vi "Delacor_lib_QMH_Error Handler - Message Handling Loop.vi"(6 "Error Message Name (\"Error\")":string="Error", 8 "error in":errorcluster, 10 "Ignore Errors (Runtime)":i32[](array[numeric]), 11 "Message Queue in":refnum<class "Delacor_lib_QMH_Message Queue.lvclass">) -> (0 "dup error in":errorcluster, 3 "Message Queue out":refnum<class "Delacor_lib_QMH_Message Queue.lvclass">)   [LabVIEW 2024, in "Delacor_lib_QMH_Message Queue.lvclass"]
doc: "Process an error that occurred in the Message Handling Loop, either by ignoring it, or generating an \"Error\" message.\n____\nDQMH Framework: Palette 7.1.0.1503\nCopyright (c) 2025, DQMH Consortium"
uses:
  Delacor_lib_QMH_Message Queue.lvclass
  Delacor_lib_QMH_Message Queue.lvclass/Delacor_lib_QMH_Message Queue.ctl
  Delacor_lib_QMH_Get Error Debug.vi
  Delacor_lib_QMH_Set Error Debug.vi
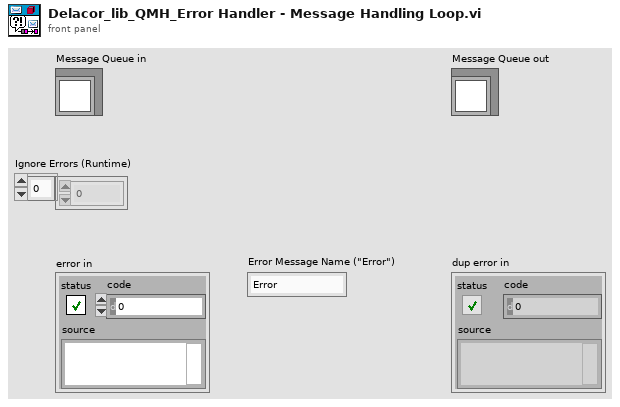
[diagram p1: front panel]
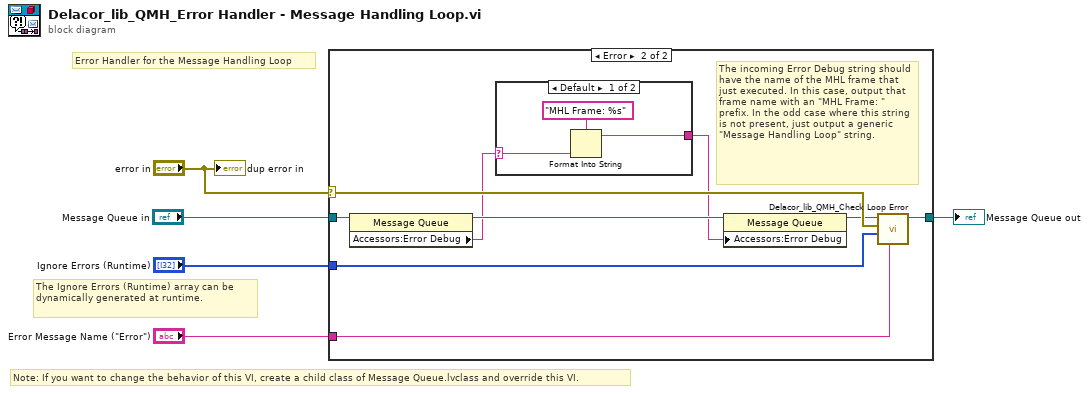
[diagram p0: block diagram]
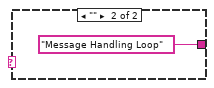
[diagram p3: hidden frame]
diagram:
  # "Note: If you want to change the behavior of this VI, create a child class of Message Queue.lvclass and override this VI."
  # "The Ignore Errors (Runtime) array can be dynamically generated at runtime."
  # "Error Handler for the Message Handling Loop"
  n1 = case shown="Error" "error in" {
    selector: "error in" -> [_ w11]
    tunnel: "Message Queue in" -> [w6 w15]
    tunnel: "Ignore Errors (Runtime)" -> [_ w14]
    tunnel: [w6 w13] -> w3
    tunnel: "Error Message Name (\"Error\")" -> [_ w12]
    frame No Error {
    }
    frame Error {
      # "The incoming Error Debug string should have the name of the MHL frame that just executed. In this case, output that frame name with an \"MHL Frame: \" prefix. In the odd case where this string is not present, just output a generic \"Message Handling Loop\" string."
      n2 = property class="Message Queue"(reference=w15) -> (reference out=w10:refnum<class "Delacor_lib_QMH_Message Queue.lvclass">, "Accessors:Error Debug"=w8:string)  [unwired: 1 in, 1 out]
      n3 = case shown="Default" w8 {
        selector: w8 -> [w18 _]
        tunnel: [w16 "Message Handling Loop"] -> w7
        frame Default {
          n4 = Format Into String(format string="MHL Frame: %s", w18) -> (resulting string=w16:string)  [unwired: 2 in, 1 out]
        }
        frame "" {
        }
      }
      n5 = property class="Message Queue"(reference=w10, "Accessors:Error Debug"=w7) -> (reference out=w9:refnum<class "Delacor_lib_QMH_Message Queue.lvclass">)  [unwired: 1 in, 1 out]
      n6 = call-dynamic "Delacor_lib_QMH_Check Loop Error.vi"("Error Message Name (\"Error\")"=w12, "Ignore Errors"=w14, "error to process"=w11, "Message Queue in"=w9) -> ("Message Queue out"=w13:refnum<class "Delacor_lib_QMH_Message Queue.lvclass">)  [unwired: 6 in, 1 out]
    }
  }
  "Message Queue out" <- w3
  "dup error in" <- "error in"
